vi "Pour.vi"(8 "error in (no error)":errorcluster, 11 "Lager in":refnum<class "Lager.lvclass">) -> (0 "error out":errorcluster, 3 "Lager out":refnum<class "Lager.lvclass">)   [LabVIEW 2011, in "Lager.lvclass"]
uses:
  Lager.lvclass
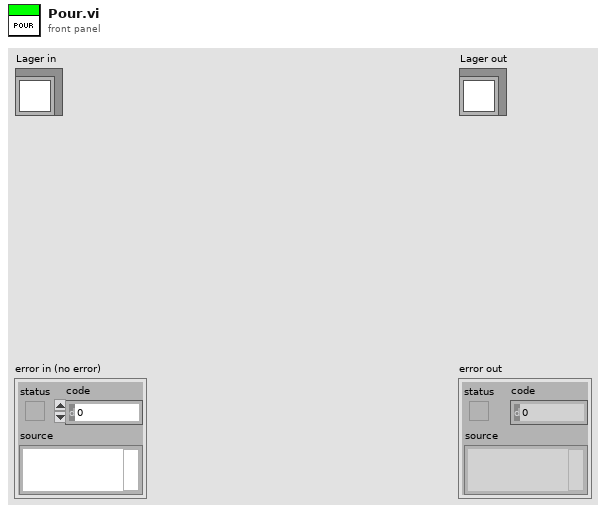
[diagram p1: front panel]
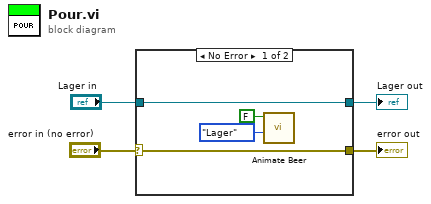
[diagram p0: block diagram]
diagram:
  n1 = case shown="No Error" "error in (no error)" {
    selector: "error in (no error)" -> [w7 w9]
    tunnel: "Lager in" -> [w8 w10]
    tunnel: [w8 w10] -> w2
    tunnel: [w7 w9] -> w1
    frame No Error {
      n2 = call "Animate Beer.vi"("Type"=enum16{"Lager", "Ale", "Guiness"}."Lager", "Tilt"=FALSE) -> ()  [unwired: 10 in]
    }
    frame Error {
    }
  }
  "error out" <- w1
  "Lager out" <- w2
